vi "Broadcast Image.vi"(8 "error in (no error)":errorcluster, 11 "Camera Process in":refnum<class "Camera Process.lvclass">) -> (0 "error out":errorcluster, 3 "Camera Process out":refnum<class "Camera Process.lvclass">)   [LabVIEW 2022 SP3, in "Cam Process.lvlib" / "Camera Process.lvclass"]
uses:
  Camera Process.lvclass
  Camera Process.lvclass/Camera Process.ctl
  Camera Data/Camera Data.lvclass/Camera Data.ctl
  Camera Data/Write Image.vi
  Camera Data/Read Events.vi
  Camera Data/Camera Data.lvclass
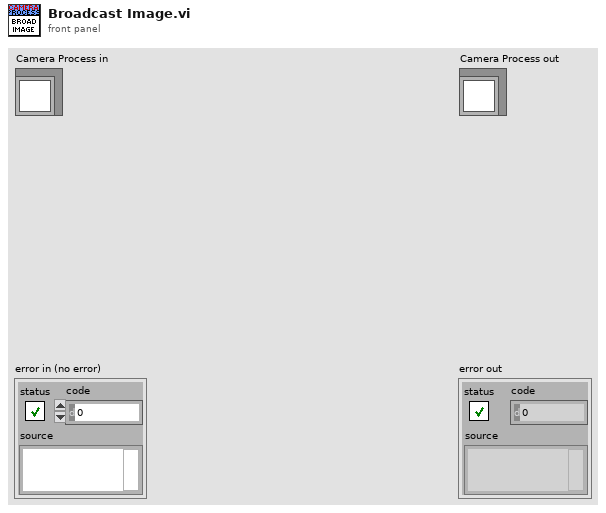
[diagram p1: front panel]
types:
  T1 = typedef "IMAQ Image.ctl" = refnum<image>
  T2 = typedef "Camera Data.lvclass/events.ctl" = cluster{"Image":refnum<user-event>}
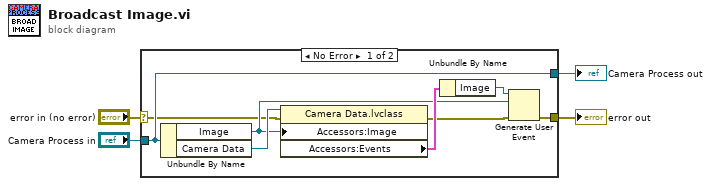
[diagram p0: block diagram]
diagram:
  n1 = case shown="No Error" "error in (no error)" {
    selector: "error in (no error)" -> [w7 w14]
    tunnel: [w5 w14] -> w3
    tunnel: [w12 w13] -> w1
    tunnel: "Camera Process in" -> [w12 w13]
    frame No Error {
      n2 = Unbundle By Name(w12) -> ("Image"=w8:T1, "Camera Data"=w11:refnum<data-value>)
      n3 = property class="Camera Data.lvclass"(reference=w11, error in=w7, "Accessors:Image"=w8) -> (error out=w6:errorcluster, "Accessors:Events"=w10:T2)  [unwired: 1 out]
      n4 = Unbundle By Name(w10) -> ("Image"=w9:refnum<user-event>)
      n5 = Generate User Event(user event=w9, event data cluster=w8, error in=w6) -> (error out=w5:errorcluster)  [unwired: 1 in, 1 out]
    }
    frame Error {
    }
  }
  "error out" <- w3
  "Camera Process out" <- w1
